vi "Enqueue Decode.vi"(8 "error in (no error)":errorcluster, 9 "Data":variant, 10 "Command":string) -> (0 "error out":errorcluster, 3 "Queue Out":T1)   [LabVIEW 2023, in "Decoder.lvlib"]
uses:
  Decoder.lvlib
  Internal Communication/Controls/Queue.ctl
  Internal Communication/Internal Communication.lvlib
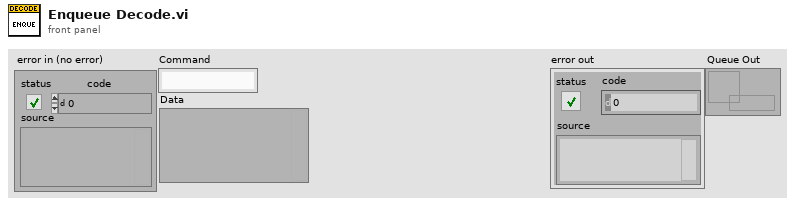
[diagram p1: front panel]
types:
  T1 = typedef "Queue.ctl" = refnum<queue>
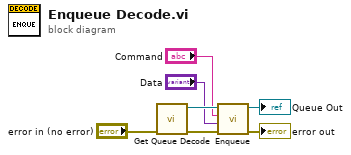
[diagram p0: block diagram]
diagram:
  n1 = call "Get Queue Decode.vi"("error in (no error)"="error in (no error)") -> ("error out"=w6:errorcluster, "Decoder Queue"=w5:refnum<queue>)  [unwired: 9 in]
  n2 = call "Enqueue.vi"("error in (no error)"=w6, "Data"="Data", "Command"="Command", "Queue In"=w5) -> ("error out"=→"error out":errorcluster, "Queue Out"=→"Queue Out":T1)  [unwired: 6 in]
